vi "parse_Testmsg.vi"(8 "error in":errorcluster, 11 "msg in":string) -> (0 "error out":errorcluster, 2 "Testmsg":T1, 3 "msg out":string)   [LabVIEW 2012]
uses:
  <userlib>/rosforlv/ROS/parsing/std_msgs/subs/parse_u8_scalar.vi
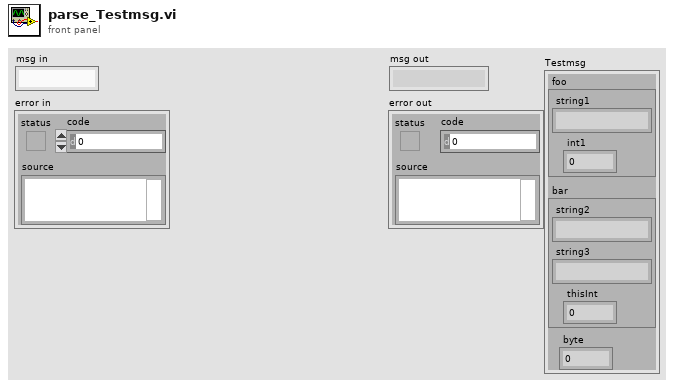
[diagram p1: front panel]
types:
  T1 = cluster{" foo":cluster{" string1":string, " int1":u32}, " bar":cluster{" string2":string, " string3":string, " thisInt":i32}, " byte":u8}
  T2 = cluster{" string2":string, " string3":string, " thisInt":i32}
  T3 = cluster{"Foo":cluster{" string1":string, " int1":u32}, "Bar":cluster{" string2":string, " string3":string, " thisInt":i32}, "number":u8}
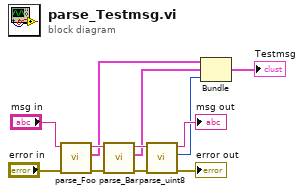
[diagram p0: block diagram]
diagram:
  n1 = call <userlib>:"parse_Foo.vi"("error in"="error in", "msg in"="msg in") -> ("error out"=w9:errorcluster, "Foo"=w4:cluster{" string1":string, " int1":u32}, "msg out"=w10:string)  [unwired: 7 in]
  n2 = call <userlib>:"parse_Bar.vi"("error in"=w9, "msg in"=w10) -> ("error out"=w7:errorcluster, "Bar"=w3:T2, "msg out"=w8:string)  [unwired: 7 in]
  n3 = call-poly <userlib>:"parse_uint8.vi"("error in"=w7, "msg in"=w8) -> ("error out"=→"error out":errorcluster, "number"=w2:u8, "msg out"=→"msg out":string)  [unwired: 3 in]
  n4 = Bundle("Foo"=w4, "Bar"=w3, "number"=w2) -> (→"Testmsg":T3)  [unwired: 1 in]
